vi "LanucherConfig.vi"   [LabVIEW 2021]
uses:
  Configuration/Top Configuration/Top Configuration.lvclass
  D:/NIO/01_Automated test platform/03_SW/02_CodeModule/01_NTP_TestSystem/01_NTP_ConfigurationAndExecution/PPL_Top/Actor Framework.lvlibp/1abvi3w/vi.lib/ActorFramework/Actor/Actor.lvclass
  PPL_Top/Actor Framework.lvlibp/1abvi3w/vi.lib/ActorFramework/Actor/Actor.lvclass
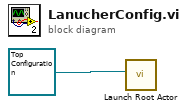
[diagram p0: block diagram]
diagram:
  n1 = call "Launch Root Actor.vi"("Actor"=refnum<class "Top Configuration.lvclass"> refnum ("Top Configuration.lvlib:Top Configuration.lvclass")) -> ()  [unwired: 9 in, 2 out]
